vi "onDisconnection.vi"(8 "error in (no error)":errorcluster, 11 "Connection.WS":refnum<class "Connection.WS.lvclass">) -> (0 "error out":errorcluster, 3 "No Connection":refnum<class "Connection.WS.lvclass">)   [LabVIEW 2013, in "Connection.WS_GOSPL.lvlib" / "Connection.WS.lvclass"]
uses:
  Connection.WS.lvclass
  Websocket Frame Type -- ring.ctl
  Connection.TCP/Connection.TCP.lvclass
  Connection/Connection.lvclass
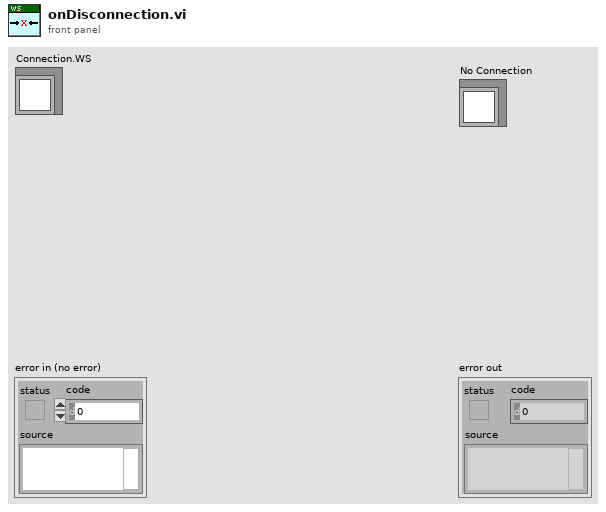
[diagram p1: front panel]
types:
  T1 = typedef "Connection.WS_GOSPL.lvlib/Connection.WS.lvclass/Websocket Frame Type -- ring.ctl" = u8
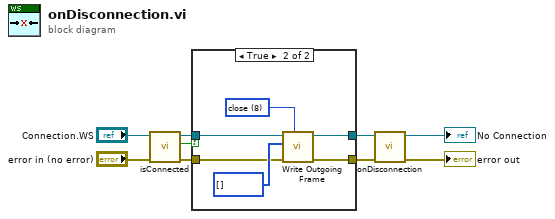
[diagram p0: block diagram]
diagram:
  n1 = call "isConnected.vi"("error in (no error)"="error in (no error)", "Connection in"="Connection.WS") -> ("error out"=w2:errorcluster, "connected"=w1:bool, "Connection out"=w4:refnum<class "Connection.WS.lvclass">)  [unwired: 7 in]
  n2 = case shown="True" w1 {
    tunnel: [w11 w17] -> w7
    tunnel: [w10 w16] -> w6
    tunnel: w4 -> [w11 w13]
    tunnel: w2 -> [w10 w12]
    frame False {
    }
    frame True {
      w15 = T1 8 items=["continuation"=0, "text"=1, "binary"=2, "close"=8, "ping"=9, "pong"=10] ("opcode")
      n3 = call "Write Outgoing Frame.vi"("Frame type"=w15, "error in (no error)"=w12, "Bytes"=u8[] [], "Connection.WS"=w13) -> ("error out"=w16:errorcluster, "Connection.WS"=w17:refnum<class "Connection.WS.lvclass">)  [unwired: 6 in]
    }
  }
  n4 = call-parent "onDisconnection.vi"("error in (no error)"=w6, "Connection.TCP"=w7) -> ("error out"=→"error out":errorcluster, "No Connection"=→"No Connection":refnum<class "Connection.WS.lvclass">)  [unwired: 8 in]
